vi "Create Transaction List.vi"(1 "Types":T3[](array[typedef]), 2 "Hold":T4, 3 "Volts":bool, 4 "Sources":T2[](array[typedef])) -> (0 "Transactions":T1[](array[typedef]))   [LabVIEW 2009]
uses:
  Apps/Yes No Button.ctl
  Dataset Type.ctl
  Dataset Source.ctl
  Dataset Transaction Id.ctl
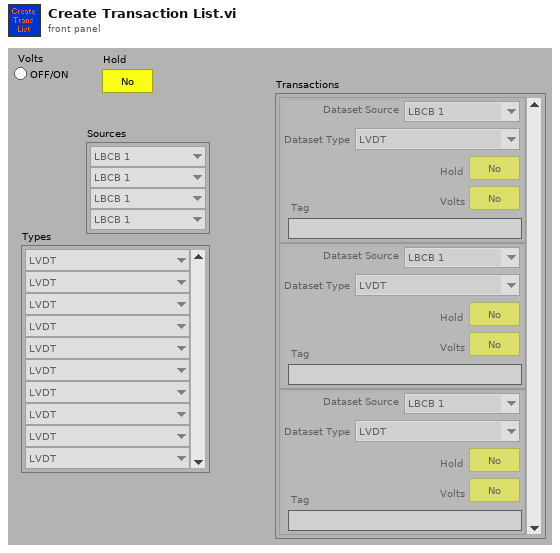
[diagram p1: front panel]
types:
  T1 = typedef "Dataset Transaction Id.ctl" = cluster{"Dataset Source":T2, "Dataset Type":T3, "Hold":T4, "Volts":T4, "Tag":string}
  T2 = typedef "Dataset Source.ctl" = enum16{"LBCB 1", "LBCB 2", "Combined", "External Sensors"}
  T3 = typedef "Dataset Type.ctl" = enum16{"LVDT", "Load Cell", "Actuator Command", "Servo Error", "Displacement Command", "Displacement", "Force"}
  T4 = typedef "Yes No Button.ctl" = bool
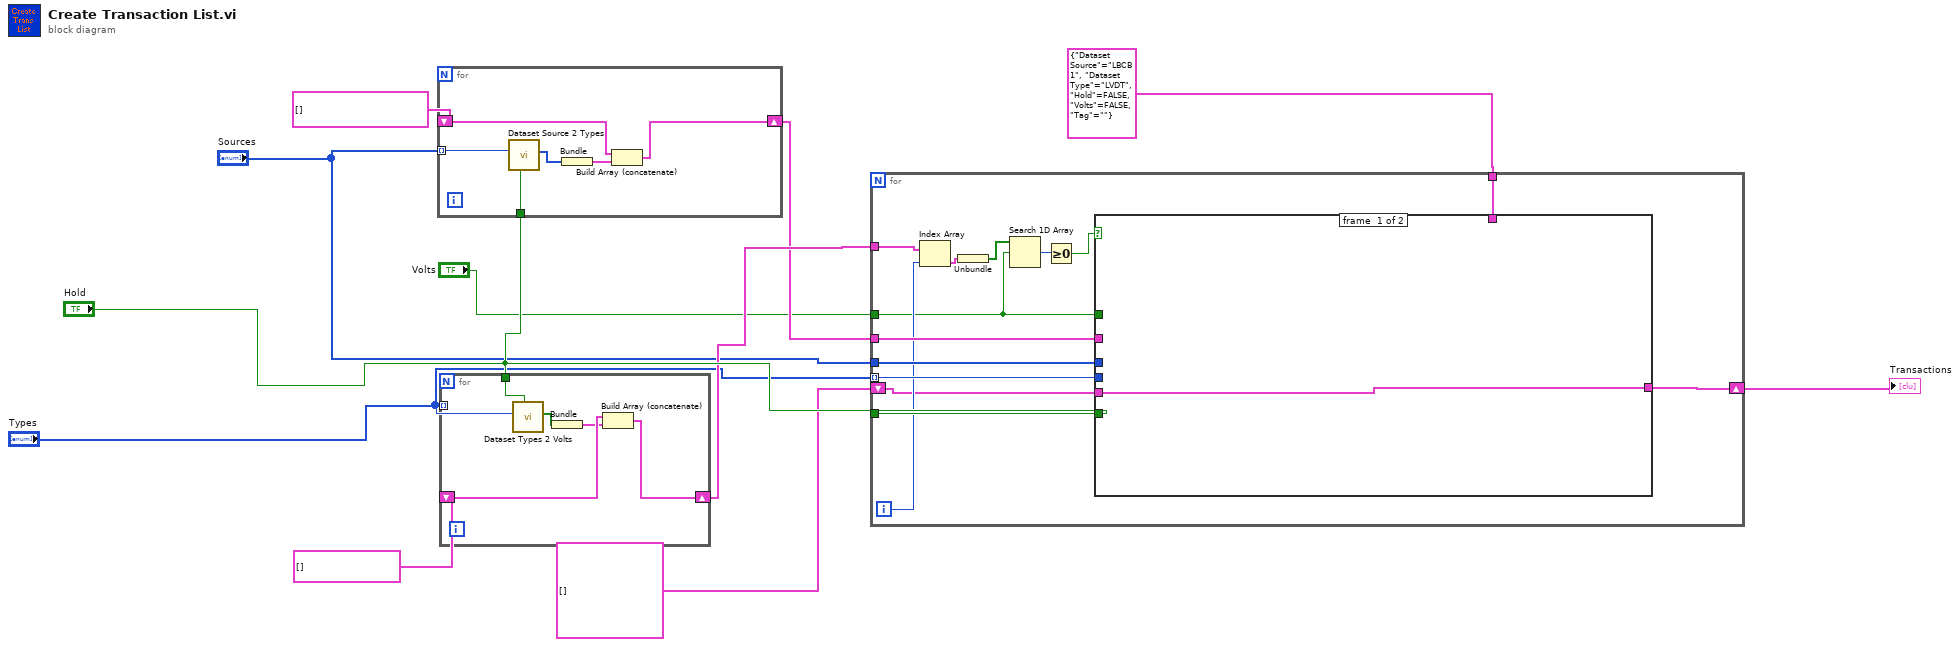
[diagram p0: block diagram]
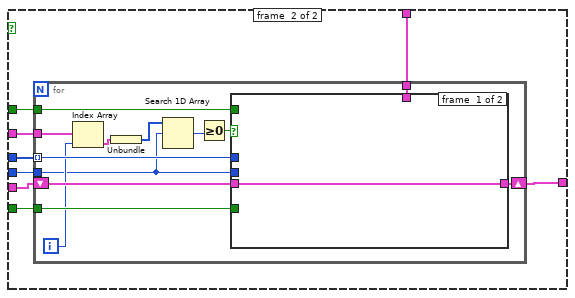
[diagram p2: hidden frame]
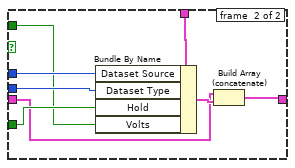
[diagram p3: hidden frame]
diagram:
  n1 = for {
    tunnel: "Sources" -> [w17] mode=indexing
    shift-right: [w16] -> w6
    shift-left: cluster{"Types":T3[]}[] [] -> [w15]
    tunnel: "Hold" -> [w12]
    n2 = call "Dataset Source 2 Types.vi"("Hold"=w12, "Dataset Source"=w17) -> ("Types"=w14:T3[])  [unwired: 9 in]
    n3 = Bundle("Types"=w14) -> (w13:cluster{"Types":T3[]})  [unwired: 1 in]
    n4 = Build Array (concatenate)(w15, w13) -> (w16:cluster{"Types":T3[]}[])
  }
  n5 = for {
    tunnel: "Types" -> [w23] mode=indexing
    shift-right: [w22] -> w7
    shift-left: cluster{"Volts Array":bool[]}[] [] -> [w21]
    tunnel: "Hold" -> [w18]
    n6 = call "Dataset Types 2 Volts.vi"("Hold"=w18, "Dataset Type"=w23) -> ("Volts Array"=w20:bool[])  [unwired: 9 in]
    n7 = Bundle("Volts Array"=w20) -> (w19:cluster{"Volts Array":bool[]})  [unwired: 1 in]
    n8 = Build Array (concatenate)(w21, w19) -> (w22:cluster{"Volts Array":bool[]}[])
  }
  n9 = for {
    tunnel: T1 {"Dataset Source"=enum."LBCB 1", "Dataset Type"=enum."LVDT", "Hold"=FALSE, "Volts"=FALSE, "Tag"=""} ("Dataset Trans Id") -> [w37]
    tunnel: "Hold" -> [w36]
    shift-right: [w24] -> w3
    shift-left: T1[] [] -> [w25]
    tunnel: "Sources" -> [w35]
    tunnel: "Types" -> [w34] mode=indexing
    tunnel: "Volts" -> [w26]
    tunnel: w6 -> [w33]
    tunnel: w7 -> [w29]
    i -> [w27]
    n10 = Index Array(array=w29, index=w27) -> (element=w32:cluster{"Volts Array":bool[]})
    n11 = Unbundle(w32) -> ("Volts Array"=w31:bool[])
    n12 = Search 1D Array(1D array=w31, element=w26) -> (index of element=w30:i32)  [unwired: 1 in]
    n13 = Greater Or Equal To 0?(x=w30) -> (x >= 0?=w28:bool)
    n14 = case shown="True" w28 {
      tunnel: w37 -> [_ w46]
      tunnel: w36 -> [_ w45]
      tunnel: [w38 w44] -> w24
      tunnel: w35 -> [_ w43]
      tunnel: w34 -> [_ w42]
      tunnel: w26 -> [_ w41]
      tunnel: w33 -> [_ w40]
      tunnel: w25 -> [w38 w39]
      frame #0 {
      }
      frame #1 {
        n15 = for {
          tunnel: w46 -> [w59]
          tunnel: w45 -> [w58]
          shift-right: [w57] -> w44
          shift-left: w39 -> [w56]
          tunnel: w43 -> [w55] mode=indexing
          tunnel: w42 -> [w47]
          tunnel: w41 -> [w54]
          tunnel: w40 -> [w53]
          i -> [w52]
          n16 = Index Array(array=w53, index=w52) -> (element=w51:cluster{"Types":T3[]})
          n17 = Unbundle(w51) -> ("Types"=w50:T3[])
          n18 = Search 1D Array(1D array=w50, element=w47) -> (index of element=w48:i32)  [unwired: 1 in]
          n19 = Greater Or Equal To 0?(x=w48) -> (x >= 0?=w49:bool)
          n20 = case shown="True" w49 {
            tunnel: w59 -> [_ w68]
            tunnel: w58 -> [_ w67]
            tunnel: [w60 w65] -> w57
            tunnel: w56 -> [w60 w64]
            tunnel: w55 -> [_ w63]
            tunnel: w47 -> [_ w62]
            tunnel: w54 -> [_ w61]
            frame #0 {
            }
            frame #1 {
              n21 = Bundle By Name(cluster=w68, "Dataset Source"=w63, "Dataset Type"=w62, "Hold"=w67, "Volts"=w61) -> (w66:T1)
              n22 = Build Array (concatenate)(w64, w66) -> (w65:T1[])
            }
          }
        }
      }
    }
  }
  "Transactions" <- w3
